vi "DeleteTestItem.vi"(1 "ModelEditInfo":T1) -> (0 "ModelEditInfo out":T1)   [LabVIEW 2014]
uses:
  ModeEditeControl.ctl
  ModelInfo.ctl
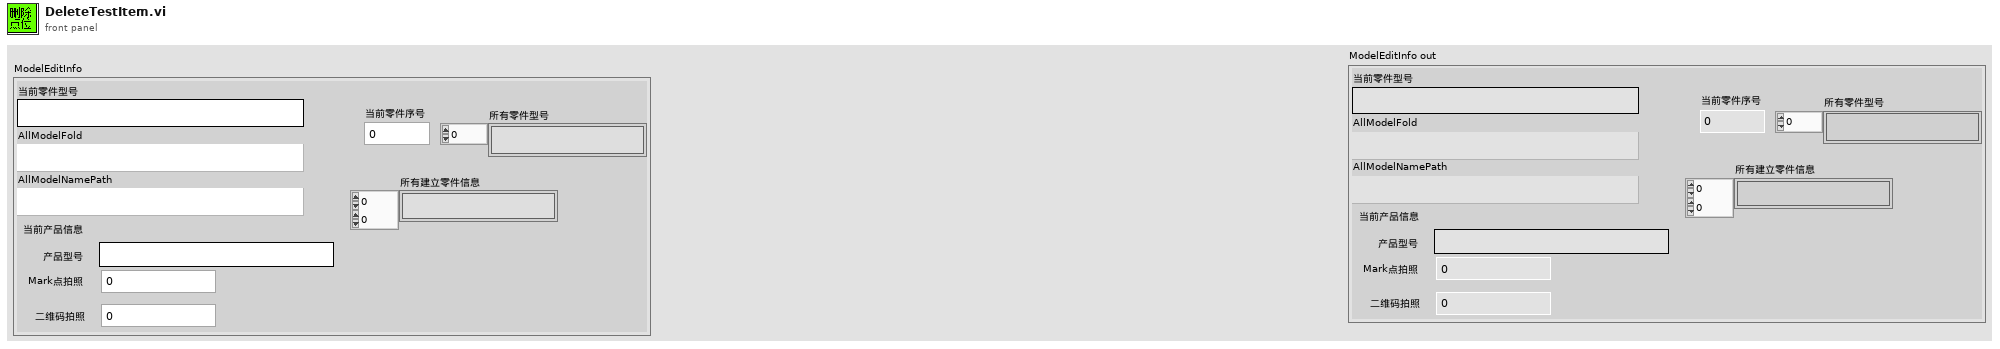
[diagram p1: front panel]
types:
  T1 = typedef "ModeEditeControl.ctl" = cluster{"AllModelFold":path, "AllModelNamePath":path, "所有零件型号":string[], "当前零件型号":string, "所有建立零件信息":string[][], "当前零件序号":i32, "当前产品信息":T2}
  T2 = typedef "ModelInfo.ctl" = cluster{"产品型号":string, "二维码拍照":u32, "Mark点拍照":u32}
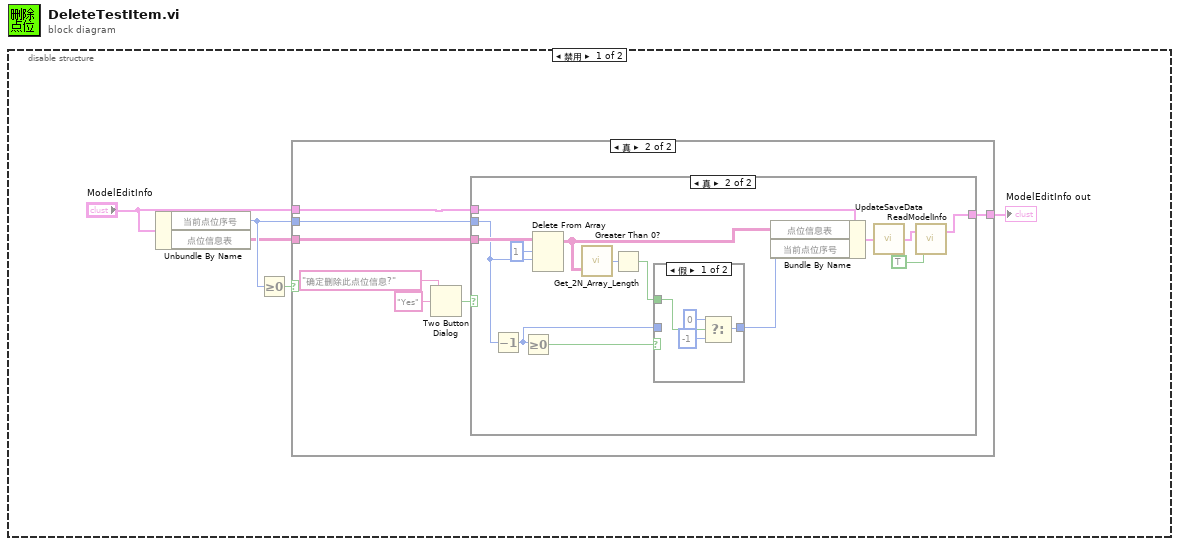
[diagram p0: block diagram]
diagram:
  n1 = disable-structure shown="禁用" {
    frame Disabled {
      n2 = Unbundle By Name("ModelEditInfo") -> ("当前点位序号"=w5:i32, "点位信息表"=w1:string[][])
      n3 = Greater Or Equal To 0?(x=w5) -> (x >= 0?=w4:bool)
      n4 = case shown="真" w4 {
        tunnel: w5 -> [_ w10]
        tunnel: w1 -> [_ w9]
        tunnel: "ModelEditInfo" -> [w6 w8]
        tunnel: [w6 w7] -> w3
        frame False {
        }
        frame True {
          n5 = Two Button Dialog(message="确定删除此点位信息?", 2:"Yes" ("T button name (\"OK\")")) -> (T button?=w11:bool)  [unwired: 1 in]
          n6 = case shown="真" w11 {
            tunnel: w9 -> [_ w27]
            tunnel: w10 -> [_ w23]
            tunnel: w8 -> [w14 w26]
            tunnel: [w14 w16] -> w7
            frame False {
            }
            frame True {
              n7 = Decrement(x=w23) -> (x-1=w18:i32)
              n8 = Greater Or Equal To 0?(x=w18) -> (x >= 0?=w24:bool)
              n9 = Delete From Array ("删除数组元素")(array=w27, length=1, index (row)=w23) -> (array with subset deleted=w21:string[][])  [unwired: 1 in, 1 out]
              n10 = call "Get_2N_Array_Length.vi"("StringArray"=w21) -> ("Numeric"=w20:i32)  [unwired: 1 in]
              n11 = Greater Than 0?(x=w20) -> (x > 0?=w19:bool)
              n12 = case shown="假" w24 {
                tunnel: w18 -> [_ w33]
                tunnel: [w29 w33] -> w22
                tunnel: w19 -> [w32 _]
                frame False {
                  n13 = Select(t=0, s=w32, f=-1) -> (s? t:f=w29:i32)
                }
                frame True {
                }
              }
              n14 = Bundle By Name(cluster=w26, "点位信息表"=w21, "当前点位序号"=w22) -> (w25:T1)
              n15 = call "UpdateSaveData.vi"("ModelEditInfo in"=w25) -> ("ModelEditInfo out"=w17:T1)
              n16 = call "ReadModelInfo.vi"("更新量测项目序号"=TRUE, "ModelEditInfo in"=w17) -> ("ModelEditInfo out"=w16:T1)  [unwired: 1 in]
            }
          }
        }
      }
      "ModelEditInfo out" <- w3
    }
    frame Enabled {
    }
  }
